vi "Get Apps.vi"(8 "error in (no error)":errorcluster, 11 "AppListPanel in":refnum<class "AppListPanel.lvclass">) -> (0 "error out":errorcluster, 2 "Apps":refnum<class "ViaApp.lvclass">[](array[class]), 3 "AppListPanel out":refnum<class "AppListPanel.lvclass">)   [LabVIEW 2020, in "PicoG-App.lvlib" / "AppListPanel.lvclass"]
uses:
  AppListPanel.lvclass
  <vilib>/IlluminatedG/IG OOPanel/OOPanel/ArrayManager/ArrayManager.lvclass
  GWebAppArrayPanel/GWebAppArrayPanel.lvclass
  ViaApp/ViaApp.lvclass
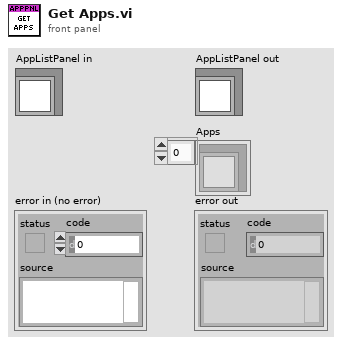
[diagram p1: front panel]
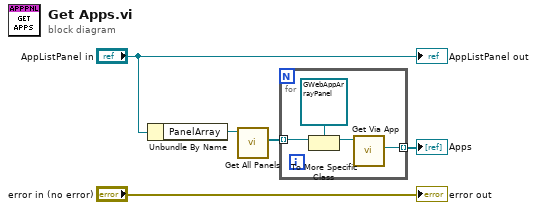
[diagram p0: block diagram]
diagram:
  n1 = Unbundle By Name("AppListPanel in") -> ("PanelArray"=w3:refnum<class "ArrayManager.lvclass">)
  n2 = call <vilib>:"Get All Panels.vi"("PanelArray in"=w3) -> ("Panels"=w2:refnum<class "ArrayPanel.lvclass">[])  [unwired: 8 in, 2 out]
  n3 = for {
    tunnel: w2 -> [w9] mode=indexing
    tunnel: [w6] -> w1 mode=indexing
    n4 = To More Specific Class(target class=refnum<class "GWebAppArrayPanel.lvclass"> refnum ("PicoG-App.lvlib:GWebAppArrayPanel.lvclass"), reference=w9) -> (specific class reference=w8:refnum<class "GWebAppArrayPanel.lvclass">)  [unwired: 1 in, 1 out]
    n5 = call "Get Via App.vi"("GWebAppArrayPanel in"=w8) -> ("App"=w6:refnum<class "ViaApp.lvclass">)  [unwired: 8 in, 2 out]
  }
  "Apps" <- w1
  "error out" <- "error in (no error)"
  "AppListPanel out" <- "AppListPanel in"
